vi "HB_ReadAISingleChannel.vi"(8 "error in (no error)":errorcluster, 10 "AI Channel":u8 max=7 step=1, 11 "HBDeviceRef":T1) -> (0 "error out":errorcluster, 1 "Raw Voltage":u32, 2 "Scaled Voltage":dbl, 3 "HBDeviceRef":T1)   [LabVIEW 2016]
doc: "Reads the specified AI channel on the Huskie Board and returns the current value both scaled and raw."
uses:
  <vilib>/Rock Robotics/WPI/SerialPort/WPI_SerialPortRef.ctl
  <vilib>/Utility/error.llb/Error Cluster From Error Code.vi
  <vilib>/ErrorRing/Error Ring.xnode
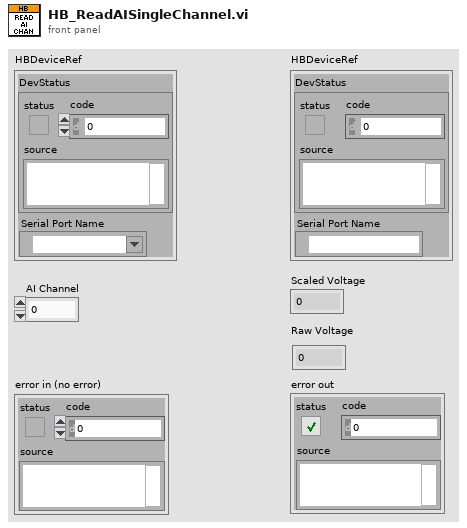
[diagram p1: front panel]
types:
  T1 = typedef "WPI_SerialPortRef.ctl" = cluster{"DevStatus":errorcluster, "Serial Port Name":refnum<visa-resource-name>}
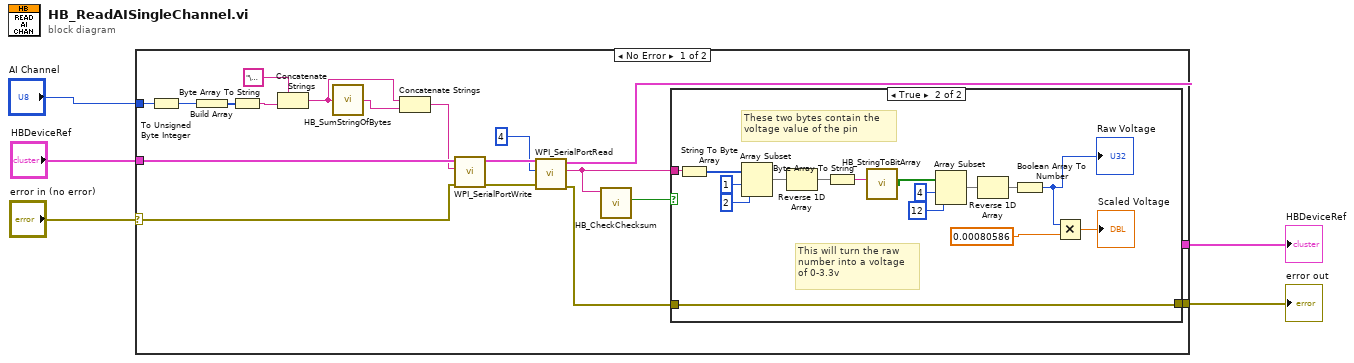
[diagram p0: block diagram]
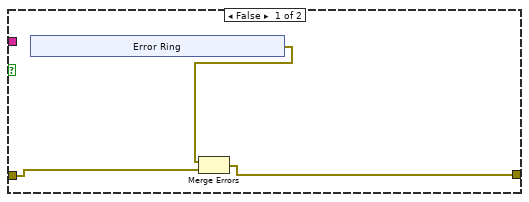
[diagram p2: hidden frame]
diagram:
  n1 = case shown="No Error" "error in (no error)" {
    selector: "error in (no error)" -> [w6 w47]
    tunnel: [w23 w47] -> w5
    tunnel: "HBDeviceRef" -> [w22 w48]
    tunnel: [w21 w48] -> w3
    tunnel: "AI Channel" -> [w7 _]
    frame No Error {
      n2 = To Unsigned Byte Integer(number=w7) -> (unsigned 8bit integer=w14:u8)
      n3 = Build Array(w14) -> (w16:u8[])
      n4 = Byte Array To String(unsigned byte array=w16) -> (string=w12:string)
      n5 = Concatenate Strings("\u0011" ("Buffer"), w12) -> (w9:string)
      n6 = call "HB_SumStringOfBytes.vi"("String Of Bytes"=w9) -> ("Sum as String"=w8:string)
      n7 = Concatenate Strings(w9, w8) -> (w15:string)
      n8 = call <vilib>:"WPI_SerialPortWrite.vi"("error in (no error)"=w6, "Buffer"=w15, "SerialPortRef"=w22) -> ("error out"=w19:errorcluster, "SerialPortRef"=w20:T1)  [unwired: 6 in, 1 out]
      n9 = call <vilib>:"WPI_SerialPortRead.vi"("error in (no error)"=w19, "Num Bytes to Read"=u32 4, "SerialPortRef"=w20) -> ("error out"=w17:errorcluster, "Buffer"=w11:string, "SerialPortRef"=w21:T1)  [unwired: 6 in]
      n10 = call "HB_CheckChecksum.vi"("String"=w11) -> ("Checksum Matches"=w10:bool)  [unwired: 9 in, 1 out]
      n11 = case shown="True" w10 {
        tunnel: w11 -> [_ w38]
        tunnel: w17 -> [w26 w37]
        tunnel: [w25 w37] -> w23
        frame False {
          n12 = xnode "Error Ring"() -> ("error out"=w24:errorcluster)
          n13 = Merge Errors(w24, w26) -> (w25:errorcluster)
        }
        frame True {
          # "This will turn the raw \nnumber into a voltage \nof 0-3.3v"
          # "These two bytes contain the \nvoltage value of the pin"
          n14 = String To Byte Array(string=w38) -> (unsigned byte array=w46:u8[])
          n15 = Array Subset(array=w46, index=1, length=2) -> (w33:u8[])
          n16 = Reverse 1D Array(array=w33) -> (reversed array=w34:u8[])
          n17 = Byte Array To String(unsigned byte array=w34) -> (string=w36:string)
          n18 = call "HB_StringToBitArray.vi"("String"=w36) -> ("Bit Array"=w35:bool[])
          n19 = Array Subset(array=w35, index=4, length=12) -> (w31:bool[])
          n20 = Reverse 1D Array(array=w31) -> (reversed array=w32:bool[])
          n21 = Boolean Array To Number(Boolean array=w32) -> (number=w41:u32)
          "Raw Voltage" <- w41
          n22 = Multiply(x=w41, y=0.00080586) -> (x*y=→"Scaled Voltage":dbl)
        }
      }
    }
    frame Error {
    }
  }
  "error out" <- w5
  "HBDeviceRef" <- w3
